vi "PathDialog.vi"(8 "error in (no error)":errorcluster, 11 "Path to Data Base in":path) -> (0 "error out":errorcluster, 3 "Path to Data Base out":path)   [LabVIEW 2015]
panel:
  in  "Set":bool
  # "Please select .db-file thats is created by EtaNet-Server. Empty paths will stopp this app and \nwrong files create errors."
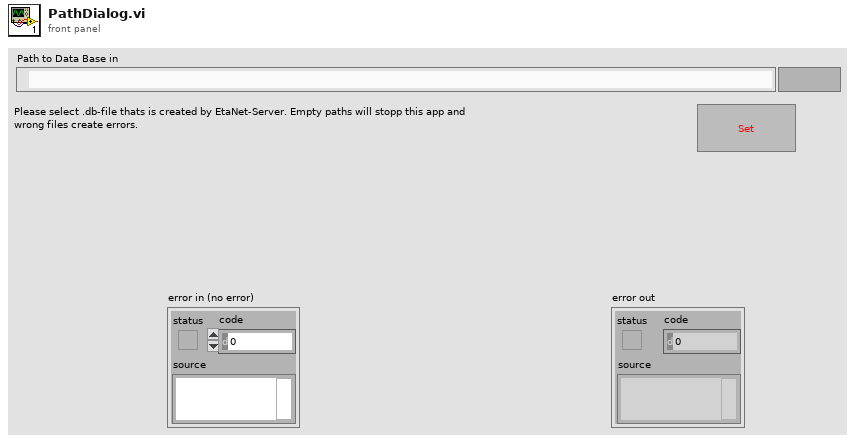
[diagram p1: front panel]
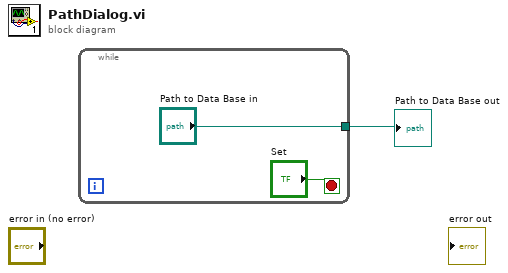
[diagram p0: block diagram]
diagram:
  n1 = while {
    tunnel: ["Path to Data Base in"] -> w1
    stop <- "Set" stop-if-true
  }
  "Path to Data Base out" <- w1
